vi "Receive Digital Inputs.vi"(8 "error in (no error)":errorcluster, 10 "Digital Input":digitalwaveform[](array[waveform]), 11 "TCP 380 in":refnum<class "TCP 380.lvclass">) -> (0 "error out":errorcluster, 3 "TCP 380 out":refnum<class "TCP 380.lvclass">)   [LabVIEW 2021, in "TCP 380.lvclass"]
uses:
  TCP 380.lvclass
  TCP 380.lvclass/TCP 380.ctl
  <vilib>/NathanCo/Digital-Tasks/Digital Input/Digital Input/Digital Input/Digital Input.lvclass
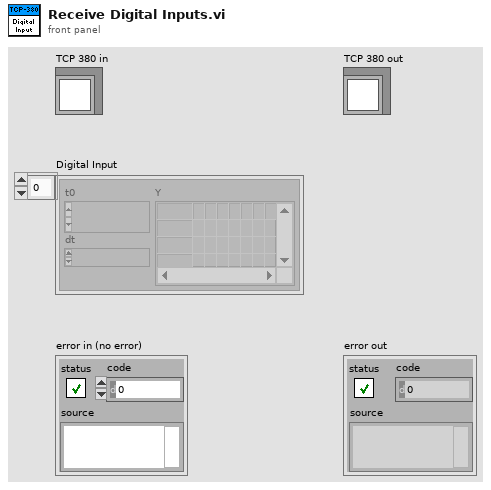
[diagram p1: front panel]
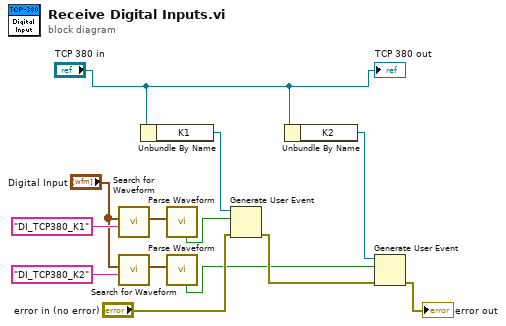
[diagram p0: block diagram]
diagram:
  n1 = call <vilib>:"Search for Waveform.vi"("NI_ChannelName"="DI_TCP380_K1" ("key"), "Waveforms"="Digital Input") -> ("Waveform"=w5:digitalwaveform)  [unwired: 8 in, 1 out]
  n2 = call <vilib>:"Search for Waveform.vi"("NI_ChannelName"="DI_TCP380_K2" ("key"), "Waveforms"="Digital Input") -> ("Waveform"=w3:digitalwaveform)  [unwired: 8 in, 1 out]
  n3 = Unbundle By Name("TCP 380 in") -> ("K1"=w13:refnum<user-event>)
  n4 = call <vilib>:"Parse Waveform.vi"("Digital Wave"=w5) -> ("Boolean"=w4:bool)  [unwired: 6 in, 4 out]
  n5 = call <vilib>:"Parse Waveform.vi"("Digital Wave"=w3) -> ("Boolean"=w2:bool)  [unwired: 6 in, 4 out]
  n6 = Generate User Event(user event=w13, event data cluster=w4, error in="error in (no error)") -> (error out=w11:errorcluster)  [unwired: 1 in, 1 out]
  n7 = Unbundle By Name("TCP 380 in") -> ("K2"=w12:refnum<user-event>)
  n8 = Generate User Event(user event=w12, event data cluster=w2, error in=w11) -> (error out=→"error out":errorcluster)  [unwired: 1 in, 1 out]
  "TCP 380 out" <- "TCP 380 in"
